vi "程序默认配置.vi"(8 "error in (no error)":errorcluster caption="错误输入（无错误）") -> (0 "error out":errorcluster caption="错误输出")   [LabVIEW 2016, in "斯坦道多参数.lvlib"]
uses:
  <vilib>/Utility/config.llb/Write Key (String).vi
  <vilib>/Utility/config.llb/NI_LVConfig.lvlib
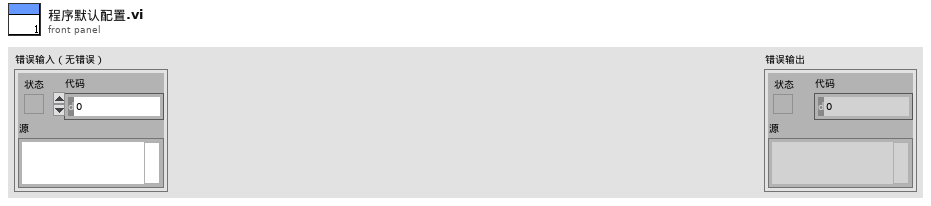
[diagram p1: front panel]
types:
  T1 = typedef "NI_LVConfig.lvlib/Config Data RefNum.ctl" = refnum<k1>
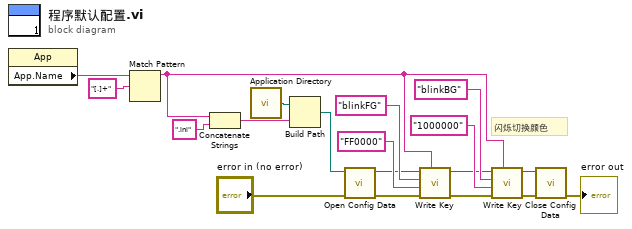
[diagram p0: block diagram]
diagram:
  # "闪烁切换颜色"
  n1 = property class="App"() -> ("App.Name"=w6:string)  [unwired: 2 in, 2 out]
  n2 = Match Pattern(string=w6, regular expression="[.]+" ("正则表达式")) -> (before substring=w15:string)  [unwired: 1 in, 3 out]
  n3 = Concatenate Strings(w15, ".ini" ("字符串")) -> (w2:string)
  n4 = call <vilib>:"Application Directory.vi"() -> ("Application Directory"=w5:path)
  n5 = Build Path(base path=w5, name or relative path=w2) -> (appended path=w8:path)
  n6 = call <vilib>:"Open Config Data.vi"("error in (no error)"="error in (no error)", "configuration file path"=w8) -> ("error out"=w10:errorcluster, "refnum"=w9:T1)  [unwired: 7 in, 1 out]
  n7 = call-poly <vilib>:"Write Key.vi"("section"=w15, "error in (no error)"=w10, "value"="FF0000" ("key"), "key"="blinkFG", "refnum"=w9) -> ("error out"=w13:errorcluster, "refnum out"=w14:T1)  [unwired: 4 in, 1 out]
  n8 = call-poly <vilib>:"Write Key.vi"("section"=w15, "error in (no error)"=w13, "value"="1000000" ("key"), "key"="blinkBG", "refnum"=w14) -> ("error out"=w18:errorcluster, "refnum out"=w19:T1)  [unwired: 4 in, 1 out]
  n9 = call <vilib>:"Close Config Data.vi"("error in (no error)"=w18, "refnum"=w19) -> ("error out"=→"error out":errorcluster)  [unwired: 8 in, 1 out]
